vi "Get Double Gyro.vi"() -> (1 "Rate":dbl, 3 "Angle":dbl)   [LabVIEW 2013]
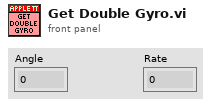
[diagram p1: front panel]
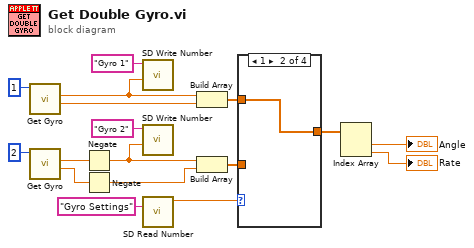
[diagram p0: block diagram]
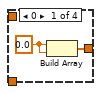
[diagram p2: hidden frame]
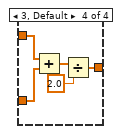
[diagram p4: hidden frame]
diagram:
  n1 = call "Get Gyro.vi"("Gyro ID (1 or 2)"=1 ("Gyro ID (0 or 1)")) -> ("Rate"=w7:dbl, "Angle"=w8:dbl)  [unwired: 9 in]
  n2 = call "Get Gyro.vi"("Gyro ID (1 or 2)"=2) -> ("Rate"=w5:dbl, "Angle"=w6:dbl)  [unwired: 9 in]
  n3 = Negate(x=w6) -> (-x=w14:dbl)
  n4 = Negate(x=w5) -> (-x=w13:dbl)
  n5 = call <vilib>:"SD Write Number.vi"("Numeric"=w8, "Name"="Gyro 1") -> ()  [unwired: 8 in, 2 out]
  n6 = call <vilib>:"SD Write Number.vi"("Numeric"=w14, "Name"="Gyro 2") -> ()  [unwired: 8 in, 2 out]
  n7 = call <vilib>:"SD Read Number.vi"("Name"="Gyro Settings") -> ("Numeric"=w17:dbl)  [unwired: 8 in, 2 out]
  n8 = Build Array(w8, w7) -> (w15:dbl[])
  n9 = Build Array(w14, w13) -> (w12:dbl[])
  n10 = case shown="1" w17 {
    tunnel: w15 -> [_ w20 _ w23]
    tunnel: w12 -> [_ _ w21 w24]
    tunnel: [w19 w20 w21 w22] -> w11
    frame 0 {
      w18 = 0.0 ("x")
      n11 = Build Array(w18, w18) -> (w19:dbl[])
    }
    frame 1 {
    }
    frame 2 {
    }
    frame 3, Default {
      n12 = Add(x=w23, y=w24) -> (x+y=w26:dbl[])
      n13 = Divide(x=w26, y=2.0) -> (x/y=w22:dbl[])
    }
  }
  n14 = Index Array(array=w11) -> (element #1=→"Angle":dbl, element #2=→"Rate":dbl)  [unwired: 2 in]
